vi "Part 2.vi"(11 "Input":string) -> (3 "Output":i64)   [LabVIEW 2021]
uses:
  a8b0d473-f658-4771-a4bf-9d8cc20f430c.vi
  <userlib>/_OpenG.lib/string/string.llb/Convert EOLs (String)__ogtk.vi
  <vilib>/Comparison/Equal/Equal Functor/Equal Functor.lvclass
panel:
  out "array":i32[][](array[numeric])
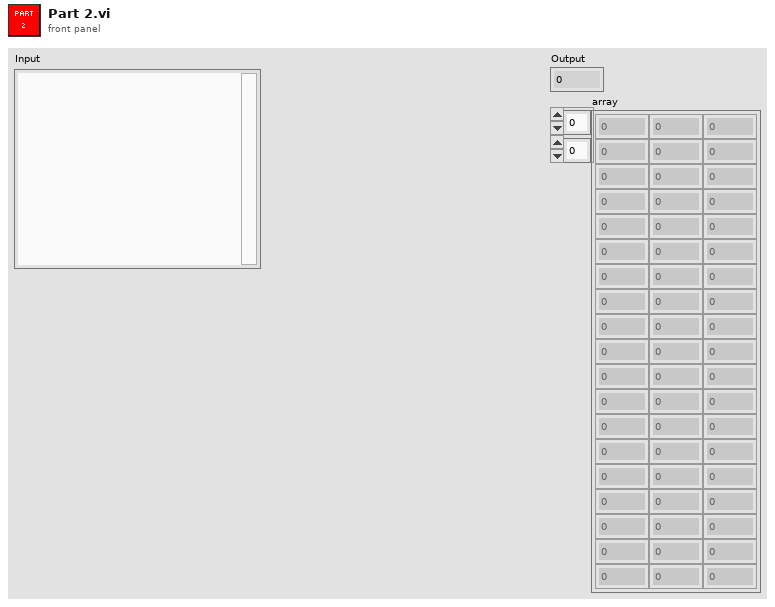
[diagram p1: front panel]
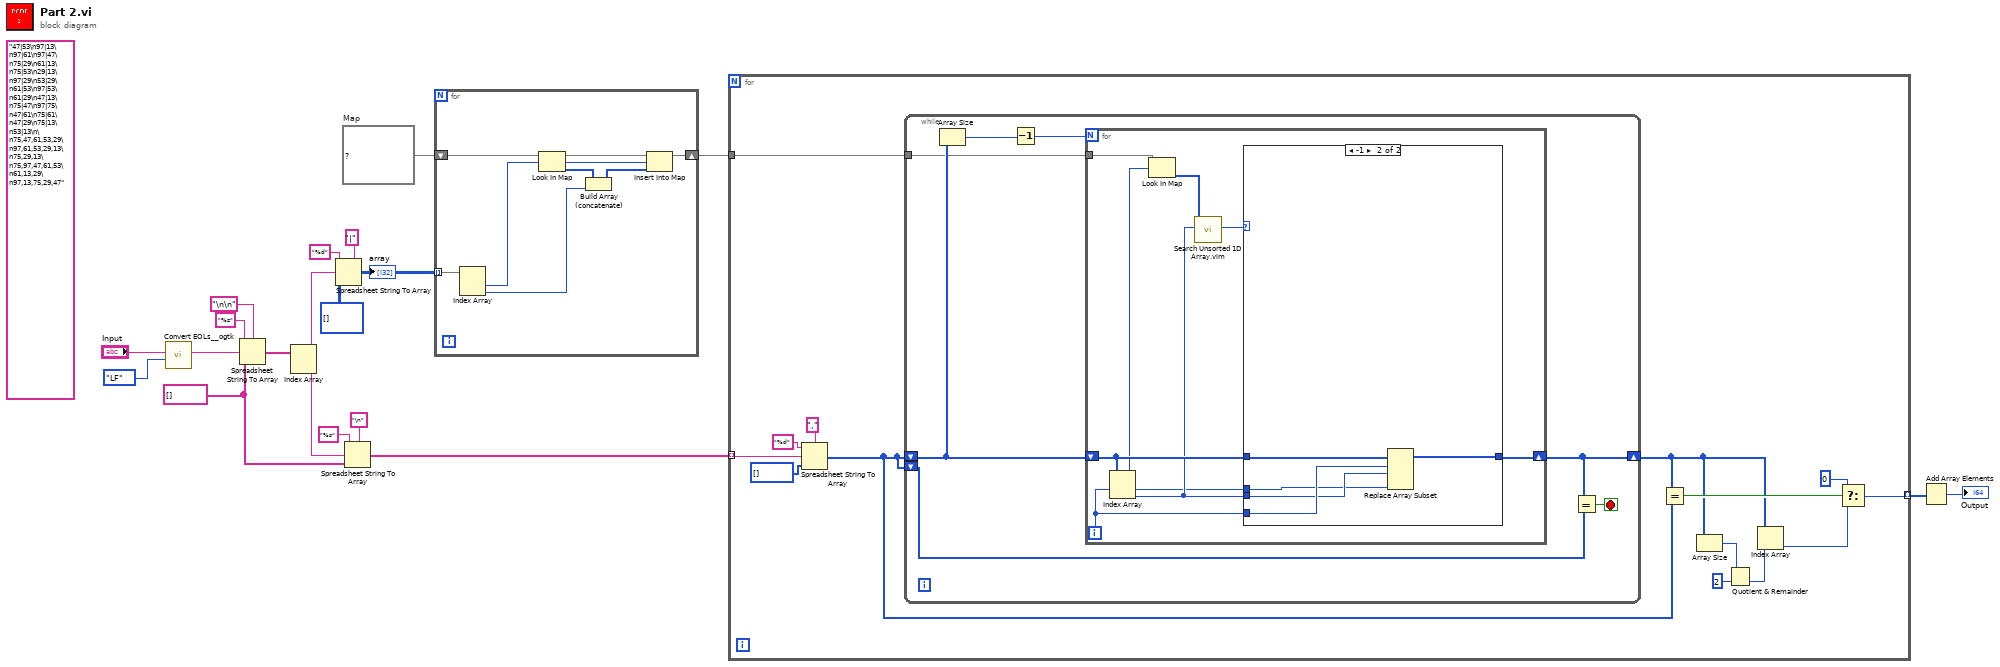
[diagram p0: block diagram]
diagram:
  w6 = map{i32, i32[]} {}  # Map
  (unwired) "47|53\n97|13\n97|61\n97|47\n75|29\n61|13\n75|53\n29|13\n97|29\n53|29\n61|53\n97|53\n61|29\n47|13\n75|47\n97|75\n47|61\n75|61\n47|29\n75|13\n53|13\n\n75,47,61,53,29\n97,61,53,29,13\n75,29,13\n75,97,47,61,53\n61,13,29\n97,13,75,29,47"
  w14 = string[] []
  n1 = call-poly <userlib>:"Convert EOLs__ogtk.vi"("Convert to:"=enum16{"CR", "LF", "CRLF"}."LF", "String in"="Input") -> ("String out"=w18:string)  [unwired: 9 in]
  n2 = Spreadsheet String To Array(delimiter (Tab)="\n\n", format string="%s", spreadsheet string=w18, array type (2D Dbl)=w14) -> (array=w16:string[])
  n3 = Index Array(array=w16) -> (element #1=w9:string, element #2=w15:string)  [unwired: 2 in]
  n4 = Spreadsheet String To Array(delimiter (Tab)="|", format string="%d", spreadsheet string=w9, array type (2D Dbl)=i32[][] []) -> (array=w7:i32[][])
  "array" <- w7
  n5 = Spreadsheet String To Array(delimiter (Tab)="\n", format string="%s", spreadsheet string=w15, array type (2D Dbl)=w14) -> (array=w4:string[])
  n6 = for {
    tunnel: w7 -> [w25] mode=indexing
    shift-right: [w27] -> w3
    shift-left: w6 -> [w26]
    n7 = Index Array(array=w25) -> (element #1=w21:i32, element #2=w22:i32)  [unwired: 2 in]
    n8 = Look In Map(map=w26, key=w21) -> (value=w24:i32[])  [unwired: 1 in, 1 out]
    n9 = Build Array (concatenate)(w24, w22) -> (w23:i32[])
    n10 = Insert Into Map(map in=w26, key=w21, value=w23) -> (map out=w27:map{i32, i32[]})  [unwired: 2 out]
  }
  n11 = for {
    tunnel: w4 -> [w38] mode=indexing
    tunnel: w3 -> [w37]
    tunnel: [w29] -> w2 mode=indexing
    n12 = Spreadsheet String To Array(delimiter (Tab)=",", format string="%d", spreadsheet string=w38, array type (2D Dbl)=i64[] []) -> (array=w28:i64[])
    n13 = while {
      shift-right: [w42] -> w34
      shift-left: w28 -> [w45]
      shift-left: w28 -> [w48]
      tunnel: w37 -> [w43]
      stop <- w47 stop-if-true
      n14 = Array Size(array=w45) -> (size(s)=w46:i32)
      n15 = Decrement(x=w46) -> (x-1=w44:i32)
      n16 = for {
        N: w44 -> [_]
        shift-right: [w52] -> w42
        shift-left: w45 -> [w54]
        tunnel: w43 -> [w56]
        i -> [w50]
        n17 = Index Array(array=w54, index #1=w50) -> (element #1=w49:i64, element #2=w51:i64)  [unwired: 1 in]
        n18 = Look In Map(map=w56, key=w49) -> (value=w55:i32[])  [unwired: 1 in, 1 out]
        n19 = call "Search Unsorted 1D Array.vim"("element"=w51, "unsorted 1D array"=w55) -> ("index of element"=w53:i32)  [unwired: 9 in]
        n20 = case shown="-1" w53 {
          tunnel: w54 -> [w57 w62]
          tunnel: [w57 w61] -> w52
          tunnel: w50 -> [_ w60]
          tunnel: w51 -> [_ w59]
          tunnel: w49 -> [_ w58]
          frame 0, Default {
          }
          frame -1 {
            n21 = Replace Array Subset(array=w62, new element #1=w59, index #1=w60, new element #2=w58) -> (w61:i64[])  [unwired: 1 in]
          }
        }
      }
      n22 = Equal?(x=w42, y=w48) -> (x = y?=w47:bool)
    }
    n23 = Equal?(x=w34, y=w28) -> (x = y?=w36:bool)
    n24 = Array Size(array=w34) -> (size(s)=w33:i32)
    n25 = Quotient & Remainder(x=w33, y=2) -> (floor(x/y)=w31:i32)  [unwired: 1 out]
    n26 = Index Array(array=w34, index=w31) -> (element=w30:i64)
    n27 = Select(t=i64 0, s=w36, f=w30) -> (s? t:f=w29:i64)
  }
  n28 = Add Array Elements(numeric array=w2) -> (sum=→"Output":i64)
